vi "User Front Panel.vi"(8 "PanelCMDRef":refnum<vi>, 10 "UserPanelCMD":refnum<queue>, 11 "PanelCluster":T1) -> ()   [LabVIEW 2020]
uses:
  <vilib>/Native 3D Graph/xcontrol/3DPC_SurfacePlot.xctl
  <vilib>/Utility/miscctls.llb/LVPointTypeDef.ctl
  CoreModules/StationModule/StationData.ctl
panel:
  in  "Tab Control":enum32{"User", "Parameter"}(tab)
  out "PathPlot":refnum<class "Base Datatype.lvclass">[](xcontrol)
  in  "Test":bool
  in  "test123":bool
  in  "ID1":bool
  in  "ID2":bool
  in  "ID3":bool
  in  "ID4":bool
  in  "ID5":bool
  in  "ID6":bool
  in  "ID7":bool
  in  "ID8":bool
  in  "ID9":bool
  in  "ID10":bool
  in  "ID12":bool
  in  "ID11":bool
  in  "LensBuffer":T2
  in  "VcmBuffer":cluster{"1":bool, "2":bool, "3":bool, "4":bool}
  in  "testtray":T3
  out "appended path":path
  in  "FeedIn":T4
  in  "FeedOut":T5
  out "Image":T6(plugin-control)
  out "Waveform":waveform(dbl)[](graph)
  out "element":T7
  in  "CRDCMPT4Y":string
  in  "CRDCMPT4X":string
  in  "CRDCMPT4Org":string
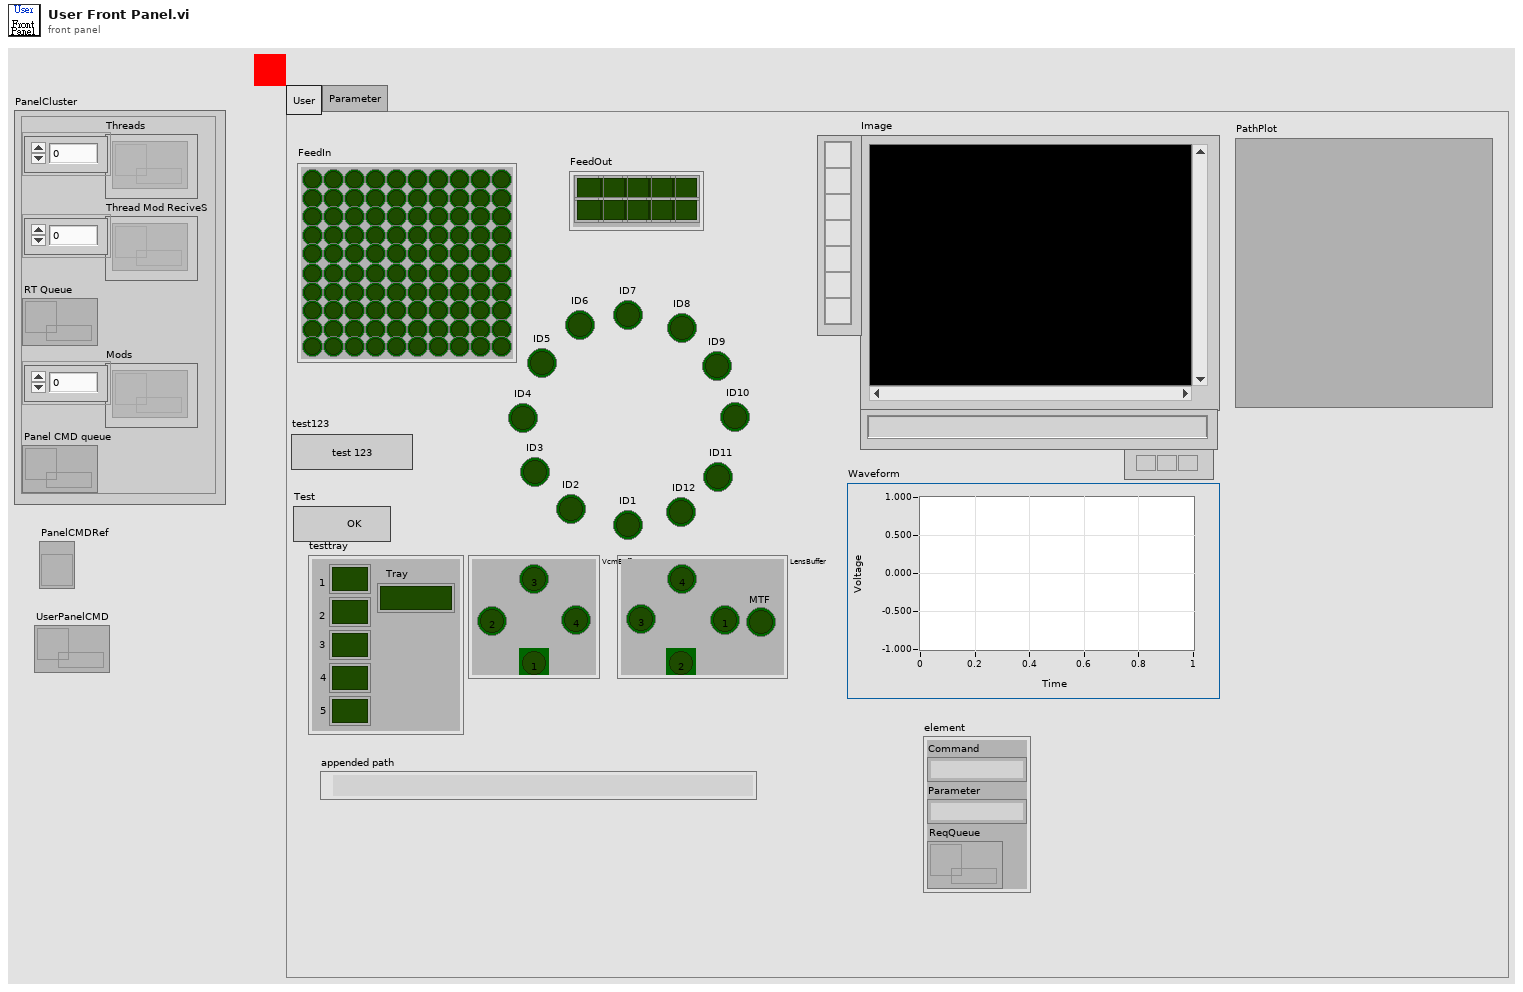
[diagram p1: front panel]
types:
  T1 = cluster{"Threads":refnum<queue>[], "Thread Mod ReciveS":refnum<queue>[], "RT Queue":refnum<queue>, "Mods":refnum<queue>[], "Panel CMD queue":refnum<queue>}
  T2 = cluster{"MTF":bool, "1":bool, "2":bool, "3":bool, "4":bool}
  T3 = cluster{"Tray":bool, "1":bool, "2":bool, "3":bool, "4":bool, "5":bool}
  T4 = cluster{"1":bool, "2":bool, "3":bool, "4":bool, "5":bool, "6":bool, "7":bool, "8":bool, "9":bool, "10":bool, "1 2":bool, "2 2":bool, "3 2":bool, "4 2":bool, "5 2":bool, "6 2":bool, "7 2":bool, "8 2":bool, "9 2":bool, "10 2":bool, "1 3":bool, "2 3":bool, "3 3":bool, "4 3":bool, "5 3":bool, "6 3":bool, "7 3":bool, "8 3":bool, "9 3":bool, "10 3":bool, "1 4":bool, "2 4":bool, "3 4":bool, "4 4":bool, "5 4":bool, "6 4":bool, "7 4":bool, "8 4":bool, "9 4":bool, "10 4":bool, "1 5":bool, "2 5":bool, "3 5":bool, "4 5":bool, "5 5":bool, "6 5":bool, "7 5":bool, "8 5":bool, "9 5":bool, "10 5":bool, "1 6":bool, "2 6":bool, "3 6":bool, "4 6":bool, "5 6":bool, "6 6":bool, "7 6":bool, "8 6":bool, "9 6":bool, "10 6":bool, "1 7":bool, "2 7":bool, "3 7":bool, "4 7":bool, "5 7":bool, "6 7":bool, "7 7":bool, "8 7":bool, "9 7":bool, "10 7":bool, "1 8":bool, "2 8":bool, "3 8":bool, "4 8":bool, "5 8":bool, "6 8":bool, "7 8":bool, "8 8":bool, "9 8":bool, "10 8":bool, "1 9":bool, "2 9":bool, "3 9":bool, "4 9":bool, "5 9":bool, "6 9":bool, "7 9":bool, "8 9":bool, "9 9":bool, "10 9":bool, "1 10":bool, "2 10":bool, "3 10":bool, "4 10":bool, "5 10":bool, "6 10":bool, "7 10":bool, "8 10":bool, "9 10":bool, "10 10":bool}
  T5 = cluster{"1":bool, "2":bool, "3":bool, "4":bool, "5":bool, "1 2":bool, "2 2":bool, "3 2":bool, "4 2":bool, "5 2":bool}
  T6 = typedef "IMAQ Image.ctl" = refnum<image>
  T7 = cluster{"Command":string, "Parameter":string, "ReqQueue":refnum<queue>}
  T8 = typedef "LVPointTypeDef.ctl" = cluster{"Horizontal":i16, "Vertical":i16}
  T9 = typedef "StationData.ctl" = enum16{"ResetDefault", "SetStationOK", "SetStationNG", "UpdateIndicator", "GetData", "SetData", "StateShift", "Init", "SetStationON", "SetStationOFF", "BlinkingON", "BlinkingOFF"}
  T10 = enum16{"Init", "AddStation", "StateShift", "ResetDefault", "SetStationON", "SetStationOFF", "SetStationOK", "SetStationNG", "UpdateIndicator", "SetData", "GetData", "GetOnOff", "GetOkNg"}
  T11 = cluster{"Program":i32, "Prog Index":i32, "State Index":i32, "State":enum16{"Init", "Idle", "Auto Start", "Auto Running", "Step Start", "Step Running", "Suspend", "Restart", "Stop", "Reset"}}
  T12 = enum16{"Get", "UpdatePointS", "Init", "UpdateIndex", "GetCurrent&Index+1", "GetWithIndex", "ChkLast", "GetCurrent"}
  T13 = cluster{"element":cluster{"Program":i32, "Prog Index":i32, "State Index":i32, "State":enum16{"Init", "Idle", "Auto Start", "Auto Running", "Step Start", "Step Running", "Suspend", "Restart", "Stop", "Reset"}}, string[][]}
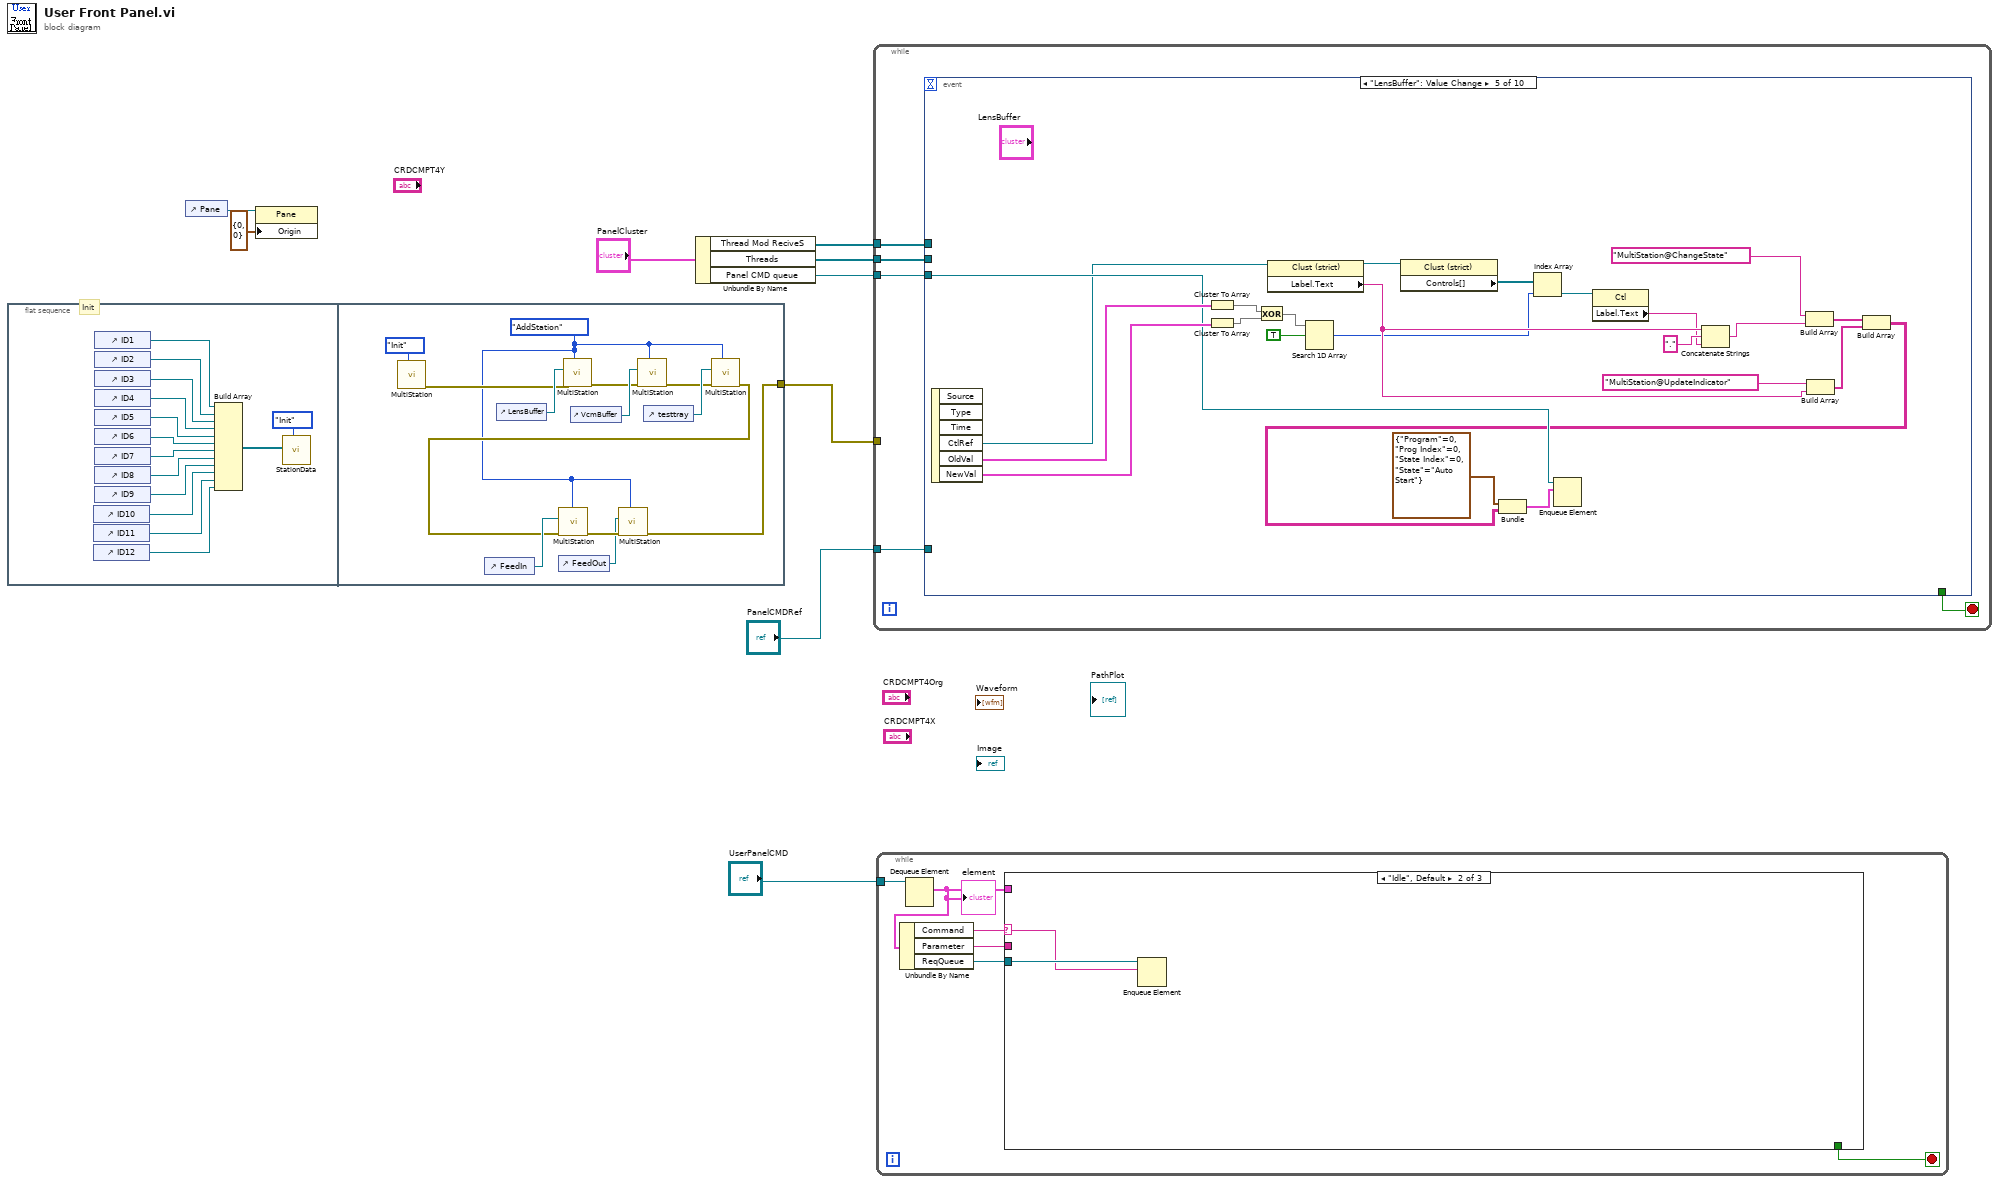
[diagram p0: block diagram]
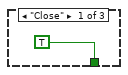
[diagram p2: hidden frame]
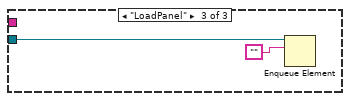
[diagram p3: hidden frame]
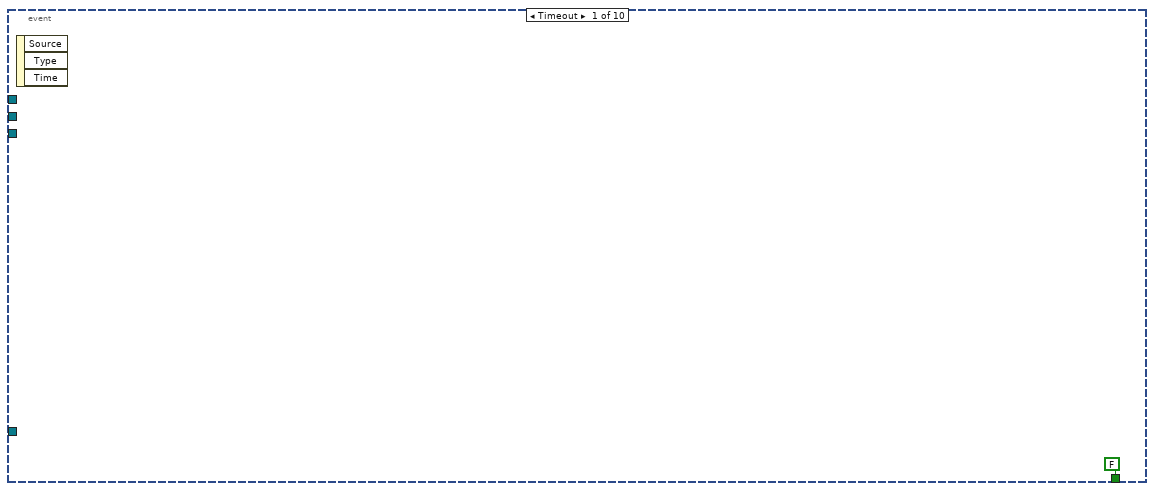
[diagram p4: hidden frame]
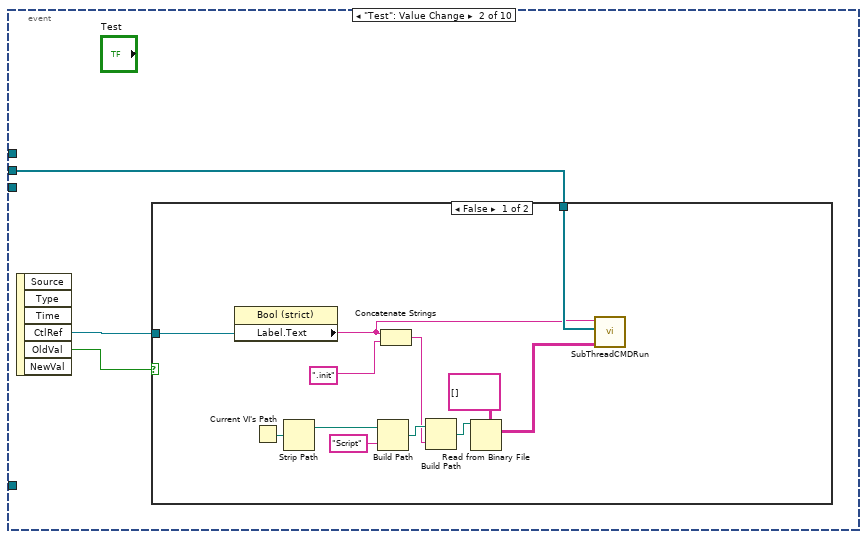
[diagram p5: hidden frame]
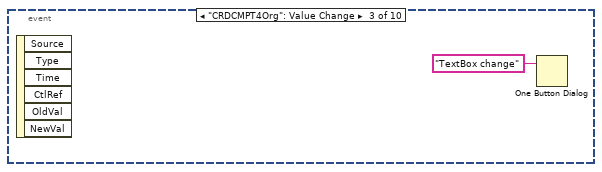
[diagram p7: hidden frame]
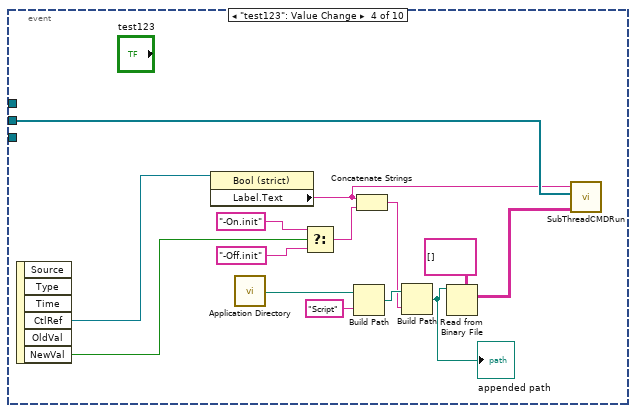
[diagram p8: hidden frame]
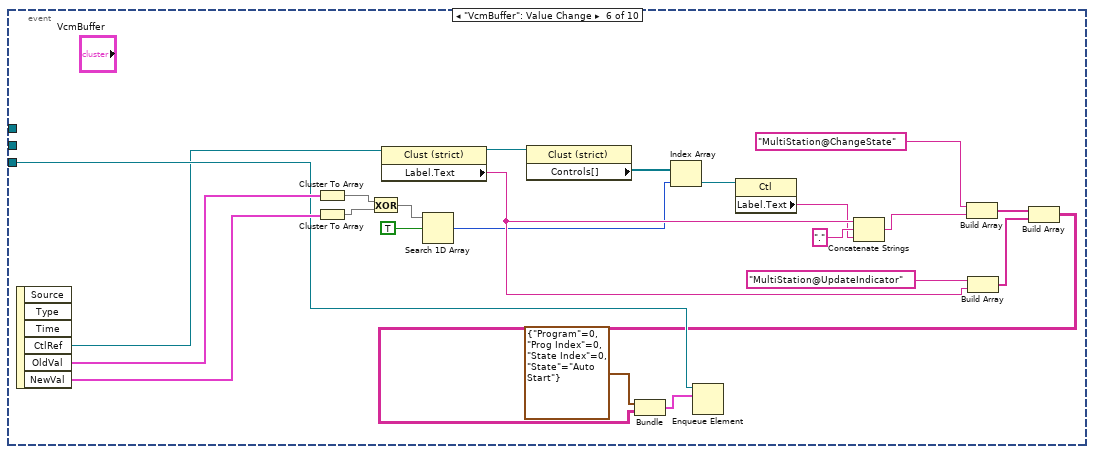
[diagram p9: hidden frame]
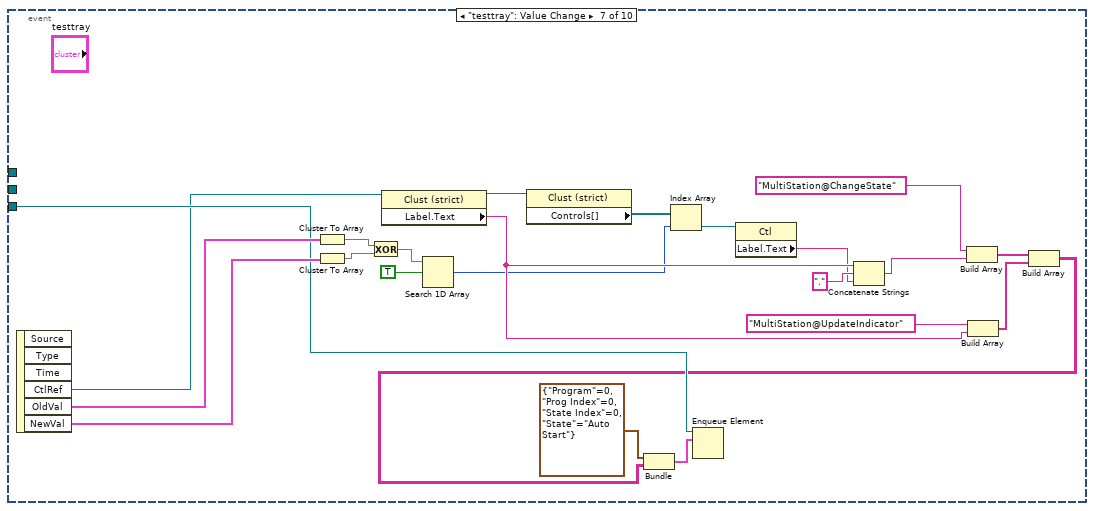
[diagram p10: hidden frame]
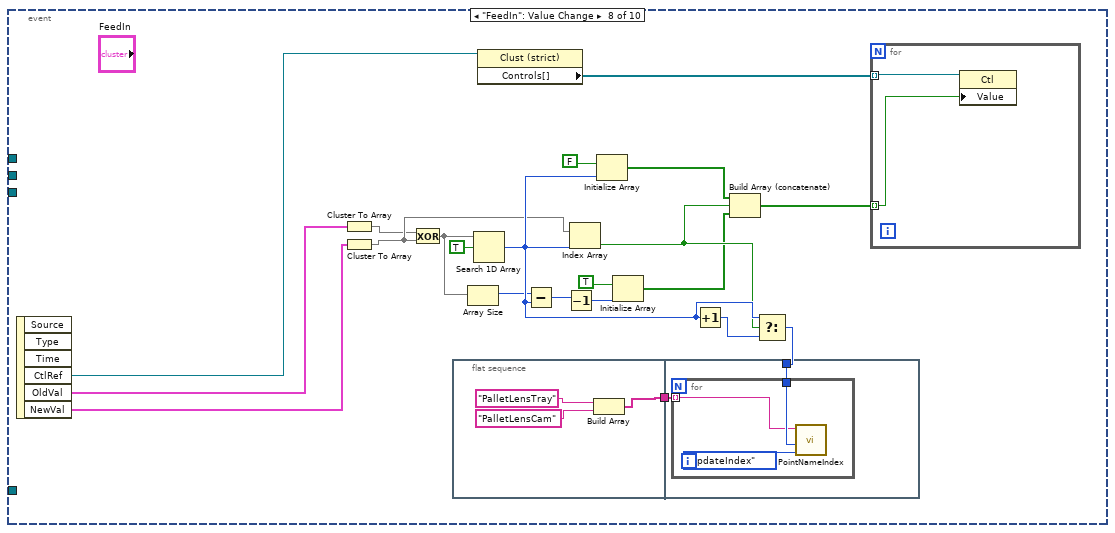
[diagram p11: hidden frame]
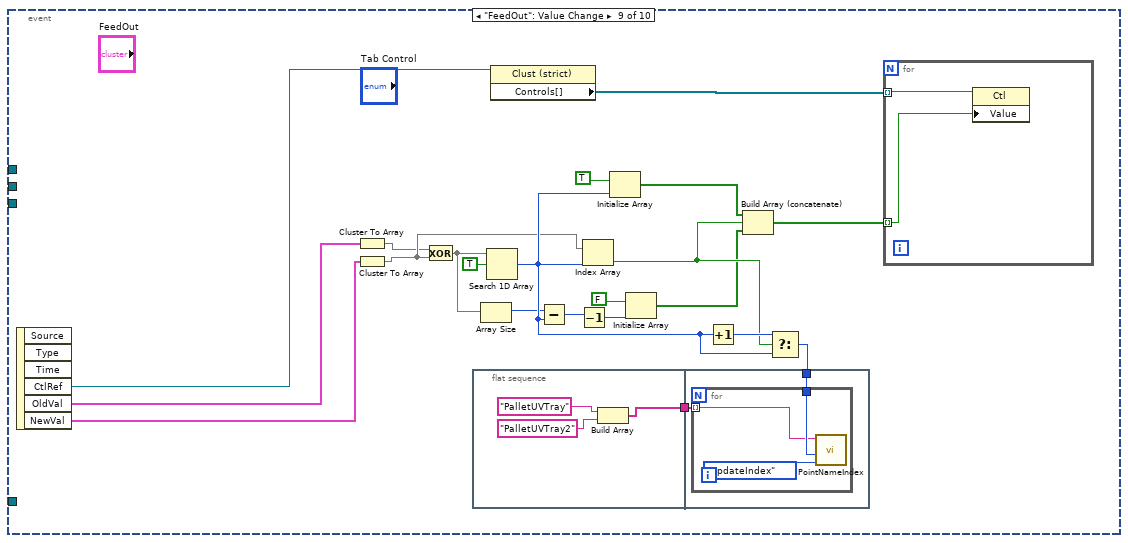
[diagram p12: hidden frame]
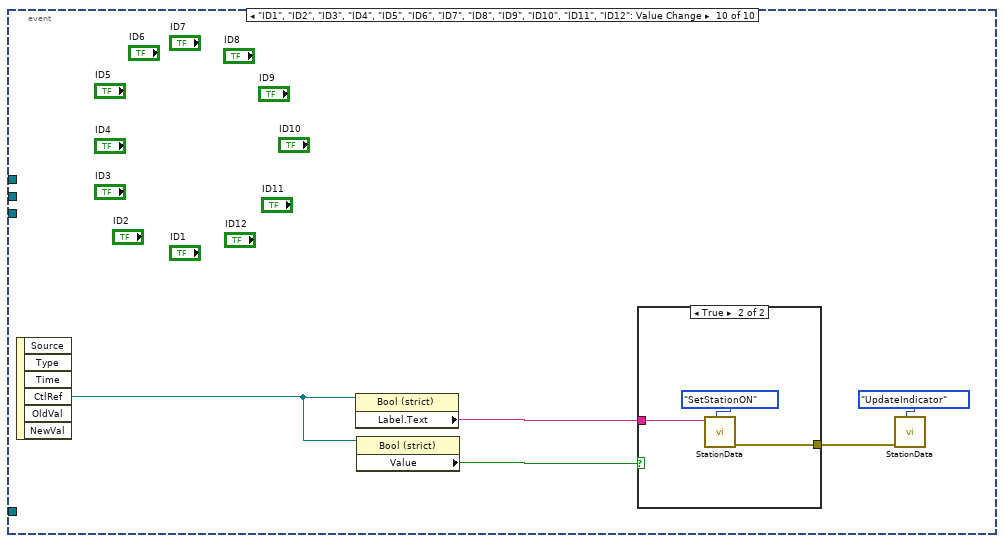
[diagram p13: hidden frame]
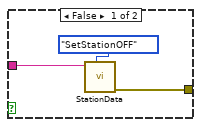
[diagram p14: hidden frame]
diagram:
  # "Init"
  n1 = flat-sequence {
    tunnel: [w25] -> w6
    frame #0 {
      n2 = control-ref of="ID10"() -> (w19:refnum<vi>)
      n3 = control-ref of="ID11"() -> (w20:refnum<vi>)
      n4 = control-ref of="ID12"() -> (w21:refnum<vi>)
      n5 = control-ref of="ID1"() -> (w10:refnum<vi>)
      n6 = control-ref of="ID2"() -> (w11:refnum<vi>)
      n7 = control-ref of="ID3"() -> (w12:refnum<vi>)
      n8 = control-ref of="ID4"() -> (w13:refnum<vi>)
      n9 = control-ref of="ID5"() -> (w14:refnum<vi>)
      n10 = control-ref of="ID6"() -> (w15:refnum<vi>)
      n11 = control-ref of="ID7"() -> (w16:refnum<vi>)
      n12 = control-ref of="ID8"() -> (w17:refnum<vi>)
      n13 = control-ref of="ID9"() -> (w18:refnum<vi>)
      n14 = Build Array(w10, w11, w12, w13, w14, w15, w16, w17, w18, w19, w20, w21) -> (w23:refnum<vi>[])
      n15 = call "StationData.vi"("CMD"=StationData."Init", "variant"=w23) -> ()  [unwired: 2 in, 8 out]
    }
    frame #1 {
      w26 = T10."AddStation" ("OP")
      n16 = call "MultiStation.vi"("OP"=T10."Init") -> ("error out"=w30:errorcluster)  [unwired: 6 in, 4 out]
      n17 = control-ref of="FeedIn"() -> (w29:refnum<vi>)
      n18 = control-ref of="LensBuffer"() -> (w36:refnum<vi>)
      n19 = control-ref of="FeedOut"() -> (w24:refnum<vi>)
      n20 = call "MultiStation.vi"("OP"=w26, "error in"=w30, "DataIn"=w36) -> ("error out"=w33:errorcluster)  [unwired: 4 in, 4 out]
      n21 = control-ref of="VcmBuffer"() -> (w35:refnum<vi>)
      n22 = call "MultiStation.vi"("OP"=w26, "error in"=w33, "DataIn"=w35) -> ("error out"=w32:errorcluster)  [unwired: 4 in, 4 out]
      n23 = control-ref of="testtray"() -> (w34:refnum<vi>)
      n24 = call "MultiStation.vi"("OP"=w26, "error in"=w32, "DataIn"=w34) -> ("error out"=w28:errorcluster)  [unwired: 4 in, 4 out]
      n25 = call "MultiStation.vi"("OP"=w26, "error in"=w28, "DataIn"=w29) -> ("error out"=w27:errorcluster)  [unwired: 4 in, 4 out]
      n26 = call "MultiStation.vi"("OP"=w26, "error in"=w27, "DataIn"=w24) -> ("error out"=w25:errorcluster)  [unwired: 4 in, 4 out]
    }
  }
  n27 = control-ref of="Pane"() -> (w2:refnum<vi>)
  n28 = property class="Pane"(reference=w2, "Origin"=T8 {"Horizontal"=0, "Vertical"=0}) -> ()  [unwired: 1 in, 2 out]
  n29 = Unbundle By Name("PanelCluster") -> ("Thread Mod ReciveS"=w9:refnum<queue>[], "Threads"=w8:refnum<queue>[], "Panel CMD queue"=w7:refnum<queue>)
  n30 = while {
    tunnel: w9 -> [w39]
    tunnel: w8 -> [w40]
    tunnel: w7 -> [w38]
    tunnel: w6 -> [_]
    tunnel: "PanelCMDRef" -> [w37]
    stop <- w41 stop-if-true
    n31 = event shown="[4] \"LensBuffer\": Value Change" {
      selector: _ -> [_ _ _ _ _ _ _ _ _ _]
      dyn-events: _ -> [_ _ _ _ _ _ _ _ _ _]
      timeout: _ -> [_ _ _ _ _ _ _ _ _ _]
      tunnel: [FALSE _ _ _ _ _ _ _ _ _] -> w41
      tunnel: w40 -> [_ w45 _ w64 _ _ _ _ _ _]
      tunnel: w39 -> [_ _ _ _ _ _ _ _ _ _]
      tunnel: w38 -> [_ _ _ _ w77 w100 w123 _ _ _]
      tunnel: w37 -> [_ _ _ _ _ _ _ _ _ _]
      event Timeout {
        n32 = event-data() -> ()  [unwired: 1 in, 3 out]
      }
      event "Test": Value Change {
        n33 = event-data() -> ("CtlRef"=w44:refnum<vi>, "OldVal"=w43:bool)  [unwired: 1 in, 4 out]
        n34 = case shown="False" w43 {
          tunnel: w45 -> [w57 _]
          tunnel: w44 -> [w56 _]
          frame False {
            n35 = property class="Bool (strict)"(reference=w56) -> ("Label.Text"=w46:string)  [unwired: 1 in, 2 out]
            n36 = Current VI's Path() -> (path=w50:path)
            n37 = Strip Path(path=w50) -> (stripped path=w49:path)  [unwired: 1 out]
            n38 = Build Path(base path=w49, name or relative path="Script") -> (appended path=w54:path)
            n39 = Concatenate Strings(w46, ".init" ("string")) -> (w53:string)
            n40 = Build Path(base path=w54, name or relative path=w53) -> (appended path=w52:path)
            n41 = Read from Binary File(5:string[][] [] ("Init Script"), 11:w52) -> (2:w48:string[][])  [unwired: 4 in, 3 out]
            n42 = call "SubThreadCMDRun.vi"("Command"=w48, "Threads"=w57, "SubThreadName"=w46) -> ()  [unwired: 8 in, 1 out]
          }
          frame True {
          }
        }
      }
      event "CRDCMPT4Org": Value Change {
        n43 = event-data() -> ()  [unwired: 1 in, 6 out]
        n44 = One Button Dialog(message="TextBox change") -> ()  [unwired: 1 in, 1 out]
      }
      event "test123": Value Change {
        n45 = event-data() -> ("CtlRef"=w63:refnum<vi>, "NewVal"=w62:bool)  [unwired: 1 in, 4 out]
        n46 = property class="Bool (strict)"(reference=w63) -> ("Label.Text"=w59:string)  [unwired: 1 in, 2 out]
        n47 = call <vilib>:"Application Directory.vi"() -> ("Application Directory"=w61:path)
        n48 = Select(t="-On.init", s=w62, f="-Off.init") -> (s? t:f=w68:string)
        n49 = Build Path(base path=w61, name or relative path="Script") -> (appended path=w71:path)
        n50 = Concatenate Strings(w59, w68) -> (w67:string)
        n51 = Build Path(base path=w71, name or relative path=w67) -> (appended path=w60:path)
        "appended path" <- w60
        n52 = Read from Binary File(5:string[][] [] ("Init Script"), 11:w60) -> (2:w65:string[][])  [unwired: 4 in, 3 out]
        n53 = call "SubThreadCMDRun.vi"("Command"=w65, "Threads"=w64, "SubThreadName"=w59) -> ()  [unwired: 8 in, 1 out]
      }
      event "LensBuffer": Value Change {
        n54 = event-data() -> ("CtlRef"=w76:refnum<vi>, "OldVal"=w79:T2, "NewVal"=w78:T2)  [unwired: 1 in, 3 out]
        n55 = Cluster To Array(cluster=w79) -> (array=w80:bool[])
        n56 = Cluster To Array(cluster=w78) -> (array=w81:bool[])
        n57 = Exclusive Or(1:w81, 2:w80) -> (0:w82:bool[])
        n58 = property class="Clust (strict)"(reference=w76) -> (reference out=w84:refnum<vi>, "Label.Text"=w94:string)  [unwired: 1 in, 1 out]
        n59 = Search 1D Array(1D array=w82, element=TRUE) -> (index of element=w86:i32)  [unwired: 1 in]
        n60 = property class="Clust (strict)"(reference=w84) -> ("Controls[]"=w85:refnum<vi>[])  [unwired: 1 in, 2 out]
        n61 = Index Array(array=w85, index=w86) -> (element=w87:refnum<vi>)
        n62 = property class="Ctl"(reference=w87) -> ("Label.Text"=w88:string)  [unwired: 1 in, 2 out]
        n63 = Concatenate Strings(w94, "." ("string"), w88) -> (w91:string)
        n64 = Build Array("MultiStation@ChangeState", w91) -> (w92:string[])
        n65 = Build Array("MultiStation@UpdateIndicator", w94) -> (w95:string[])
        n66 = Build Array(w92, w95) -> (w74:string[][])
        n67 = Bundle("element"=T11 {"Program"=0, "Prog Index"=0, "State Index"=0, "State"=enum."Auto Start"}, w74) -> (w73:T13)  [unwired: 1 in]
        n68 = Enqueue Element(queue=w77, element=w73) -> ()  [unwired: 1 in, 4 out]
      }
      event "VcmBuffer": Value Change {
        n69 = event-data() -> ("CtlRef"=w99:refnum<vi>, "OldVal"=w102:cluster{"1":bool, "2":bool, "3":bool, "4":bool}, "NewVal"=w101:cluster{"1":bool, "2":bool, "3":bool, "4":bool})  [unwired: 1 in, 3 out]
        n70 = Cluster To Array(cluster=w102) -> (array=w103:bool[])
        n71 = Cluster To Array(cluster=w101) -> (array=w104:bool[])
        n72 = Exclusive Or(1:w104, 2:w103) -> (0:w105:bool[])
        n73 = property class="Clust (strict)"(reference=w99) -> (reference out=w107:refnum<vi>, "Label.Text"=w117:string)  [unwired: 1 in, 1 out]
        n74 = Search 1D Array(1D array=w105, element=TRUE) -> (index of element=w109:i32)  [unwired: 1 in]
        n75 = property class="Clust (strict)"(reference=w107) -> ("Controls[]"=w108:refnum<vi>[])  [unwired: 1 in, 2 out]
        n76 = Index Array(array=w108, index=w109) -> (element=w110:refnum<vi>)
        n77 = property class="Ctl"(reference=w110) -> ("Label.Text"=w111:string)  [unwired: 1 in, 2 out]
        n78 = Concatenate Strings(w117, "." ("string"), w111) -> (w114:string)
        n79 = Build Array("MultiStation@ChangeState", w114) -> (w115:string[])
        n80 = Build Array("MultiStation@UpdateIndicator", w117) -> (w118:string[])
        n81 = Build Array(w115, w118) -> (w97:string[][])
        n82 = Bundle("element"=T11 {"Program"=0, "Prog Index"=0, "State Index"=0, "State"=enum."Auto Start"}, w97) -> (w96:T13)  [unwired: 1 in]
        n83 = Enqueue Element(queue=w100, element=w96) -> ()  [unwired: 1 in, 4 out]
      }
      event "testtray": Value Change {
        n84 = event-data() -> ("CtlRef"=w122:refnum<vi>, "OldVal"=w125:T3, "NewVal"=w124:T3)  [unwired: 1 in, 3 out]
        n85 = Cluster To Array(cluster=w125) -> (array=w126:bool[])
        n86 = Cluster To Array(cluster=w124) -> (array=w127:bool[])
        n87 = Exclusive Or(1:w127, 2:w126) -> (0:w128:bool[])
        n88 = property class="Clust (strict)"(reference=w122) -> (reference out=w130:refnum<vi>, "Label.Text"=w140:string)  [unwired: 1 in, 1 out]
        n89 = Search 1D Array(1D array=w128, element=TRUE) -> (index of element=w132:i32)  [unwired: 1 in]
        n90 = property class="Clust (strict)"(reference=w130) -> ("Controls[]"=w131:refnum<vi>[])  [unwired: 1 in, 2 out]
        n91 = Index Array(array=w131, index=w132) -> (element=w133:refnum<vi>)
        n92 = property class="Ctl"(reference=w133) -> ("Label.Text"=w134:string)  [unwired: 1 in, 2 out]
        n93 = Concatenate Strings(w140, "." ("string"), w134) -> (w137:string)
        n94 = Build Array("MultiStation@ChangeState", w137) -> (w138:string[])
        n95 = Build Array("MultiStation@UpdateIndicator", w140) -> (w141:string[])
        n96 = Build Array(w138, w141) -> (w120:string[][])
        n97 = Bundle("element"=T11 {"Program"=0, "Prog Index"=0, "State Index"=0, "State"=enum."Auto Start"}, w120) -> (w119:T13)  [unwired: 1 in]
        n98 = Enqueue Element(queue=w123, element=w119) -> ()  [unwired: 1 in, 4 out]
      }
      event "FeedIn": Value Change {
        n99 = event-data() -> ("CtlRef"=w144:refnum<vi>, "OldVal"=w143:T4, "NewVal"=w142:T4)  [unwired: 1 in, 3 out]
        n100 = Cluster To Array(cluster=w143) -> (array=w145:bool[])
        n101 = Cluster To Array(cluster=w142) -> (array=w155:bool[])
        n102 = Exclusive Or(1:w155, 2:w145) -> (0:w148:bool[])
        n103 = flat-sequence {
          tunnel: [w163] -> w162
          tunnel: w159 -> [w167]
          tunnel: w162 -> [w166]
          frame #0 {
            n104 = Build Array("PalletLensTray", "PalletLensCam") -> (w163:string[])
          }
          frame #1 {
            n105 = for {
              tunnel: w167 -> [w170]
              tunnel: w166 -> [w169] mode=indexing
              n106 = call "PointNameIndex.vi"("OP"=T12."UpdateIndex", "PathIndexIn"=w170, "PointName"=w169) -> ()  [unwired: 3 in, 6 out]
            }
          }
        }
        n107 = Array Size(array=w148) -> (size(s)=w149:i32)
        n108 = Search 1D Array(1D array=w148, element=TRUE) -> (index of element=w161:i32)  [unwired: 1 in]
        n109 = property class="Clust (strict)"(reference=w144) -> ("Controls[]"=w156:refnum<vi>[])  [unwired: 1 in, 2 out]
        n110 = Subtract(x=w149, y=w161) -> (x-y=w153:i32)
        n111 = Decrement(x=w153) -> (x-1=w154:i32)
        n112 = Index Array(array=w155, index=w161) -> (element=w158:bool)
        n113 = Initialize Array(FALSE ("element"), w161) -> (w151:bool[])
        n114 = Initialize Array(TRUE ("element"), w154) -> (w152:bool[])
        n115 = Increment(x=w161) -> (x+1=w160:i32)
        n116 = Build Array (concatenate)(w151, w158, w152) -> (w157:bool[])
        n117 = Select(t=w161, s=w158, f=w160) -> (s? t:f=w159:i32)
        n118 = for {
          tunnel: w156 -> [w172] mode=indexing
          tunnel: w157 -> [w171] mode=indexing
          n119 = property class="Ctl"(reference=w172, "Value"=w171) -> ()  [unwired: 1 in, 2 out]
        }
      }
      event "FeedOut": Value Change {
        n120 = event-data() -> ("CtlRef"=w175:refnum<vi>, "OldVal"=w174:T5, "NewVal"=w173:T5)  [unwired: 1 in, 3 out]
        n121 = Cluster To Array(cluster=w174) -> (array=w176:bool[])
        n122 = Cluster To Array(cluster=w173) -> (array=w186:bool[])
        n123 = Exclusive Or(1:w186, 2:w176) -> (0:w179:bool[])
        n124 = flat-sequence {
          tunnel: [w194] -> w193
          tunnel: w190 -> [w198]
          tunnel: w193 -> [w197]
          frame #0 {
            n125 = Build Array("PalletUVTray", "PalletUVTray2") -> (w194:string[])
          }
          frame #1 {
            n126 = for {
              tunnel: w198 -> [w201]
              tunnel: w197 -> [w200] mode=indexing
              n127 = call "PointNameIndex.vi"("OP"=T12."UpdateIndex", "PathIndexIn"=w201, "PointName"=w200) -> ()  [unwired: 3 in, 6 out]
            }
          }
        }
        n128 = Array Size(array=w179) -> (size(s)=w180:i32)
        n129 = Search 1D Array(1D array=w179, element=TRUE) -> (index of element=w192:i32)  [unwired: 1 in]
        n130 = property class="Clust (strict)"(reference=w175) -> ("Controls[]"=w187:refnum<vi>[])  [unwired: 1 in, 2 out]
        n131 = Subtract(x=w180, y=w192) -> (x-y=w184:i32)
        n132 = Decrement(x=w184) -> (x-1=w185:i32)
        n133 = Index Array(array=w186, index=w192) -> (element=w189:bool)
        n134 = Initialize Array(TRUE ("element"), w192) -> (w182:bool[])
        n135 = Initialize Array(FALSE ("element"), w185) -> (w183:bool[])
        n136 = Increment(x=w192) -> (x+1=w191:i32)
        n137 = Build Array (concatenate)(w182, w189, w183) -> (w188:bool[])
        n138 = Select(t=w191, s=w189, f=w192) -> (s? t:f=w190:i32)
        n139 = for {
          tunnel: w187 -> [w203] mode=indexing
          tunnel: w188 -> [w202] mode=indexing
          n140 = property class="Ctl"(reference=w203, "Value"=w202) -> ()  [unwired: 1 in, 2 out]
        }
      }
      event "ID1", "ID2", "ID3", "ID4", "ID5", "ID6", "ID7", "ID8", "ID9", "ID10", "ID11", "ID12": Value Change {
        n141 = event-data() -> ("CtlRef"=w204:refnum<vi>)  [unwired: 1 in, 5 out]
        n142 = property class="Bool (strict)"(reference=w204) -> ("Label.Text"=w206:string)  [unwired: 1 in, 2 out]
        n143 = property class="Bool (strict)"(reference=w204) -> ("Value"=w205:bool)  [unwired: 1 in, 2 out]
        n144 = case shown="True" w205 {
          tunnel: w206 -> [w210 w213]
          tunnel: [w209 w212] -> w208
          frame False {
            n145 = call "StationData.vi"("CMD"=StationData."SetStationOFF", "StationID"=w210) -> ("error out"=w209:errorcluster)  [unwired: 2 in, 7 out]
          }
          frame True {
            n146 = call "StationData.vi"("CMD"=StationData."SetStationON", "StationID"=w213) -> ("error out"=w212:errorcluster)  [unwired: 2 in, 7 out]
          }
        }
        n147 = call "StationData.vi"("CMD"=StationData."UpdateIndicator", "error in"=w208) -> ()  [unwired: 2 in, 8 out]
      }
    }
  }
  n148 = while {
    tunnel: "UserPanelCMD" -> [w220]
    stop <- w219 stop-if-true
    n149 = Dequeue Element(queue=w220) -> (element=w217:T7)  [unwired: 2 in, 3 out]
    "element" <- w217
    n150 = Unbundle By Name(w217) -> ("Command"=w218:string, "Parameter"=w215:string, "ReqQueue"=w216:refnum<queue>)
    n151 = case shown="\"Idle\", Default" w218 {
      selector: w218 -> [_ w222 _]
      tunnel: [TRUE _ _] -> w219
      tunnel: w217 -> [_ _ _]
      tunnel: w216 -> [_ w223 w224]
      tunnel: w215 -> [_ _ _]
      frame "Close" {
      }
      frame "Idle", Default {
        n152 = Enqueue Element(queue=w223, element=w222) -> ()  [unwired: 2 in, 3 out]
      }
      frame "LoadPanel" {
        n153 = Enqueue Element(queue=w224, element="") -> ()  [unwired: 2 in, 3 out]
      }
    }
  }
